vi "set offset.vi"(8 "error in (no error)":errorcluster, 11 "Thorcam in":refnum<class "Thorcam.lvclass">) -> (0 "error out":errorcluster, 3 "Thorcam out":refnum<class "Thorcam.lvclass">)   [LabVIEW 2012, in "Thorcam.lvclass"]
uses:
  Thorcam.lvclass
  Thorcam.lvclass/Thorcam.ctl
panel:
  out "Value":i32
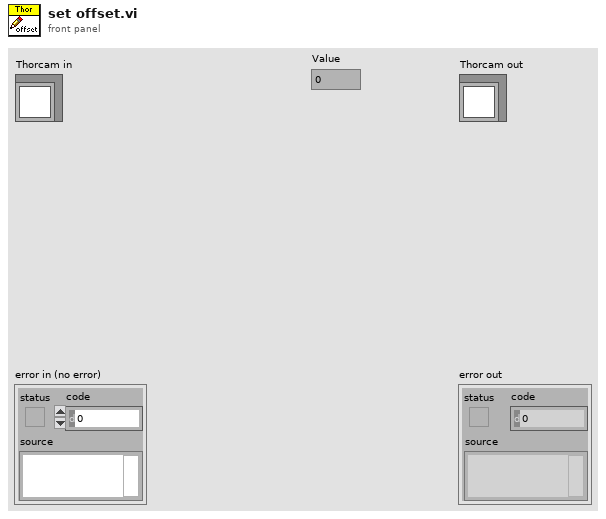
[diagram p1: front panel]
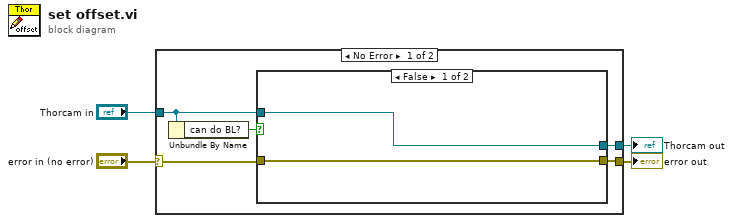
[diagram p0: block diagram]
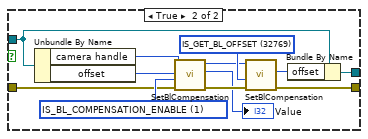
[diagram p2: hidden frame]
diagram:
  n1 = case shown="No Error" "error in (no error)" {
    selector: "error in (no error)" -> [w9 w25]
    tunnel: [w6 w25] -> w3
    tunnel: [w5 w24] -> w1
    tunnel: "Thorcam in" -> [w8 w24]
    frame No Error {
      n2 = Unbundle By Name(w8) -> ("can do BL?"=w7:bool)
      n3 = case shown="False" w7 {
        tunnel: w8 -> [w11 w14]
        tunnel: w9 -> [w10 w21]
        tunnel: [w10 w18] -> w6
        tunnel: [w11 w13] -> w5
        frame False {
        }
        frame True {
          w17 = 32769 items=["IS_BL_COMPENSATION_DISABLE"=0, "IS_BL_COMPENSATION_ENABLE"=1, "IS_GET_BL_COMPENSATION"=32768, "IS_GET_BL_OFFSET"=32769, "IS_GET_BL_DEFAULT_MODE"=32770, "IS_GET_BL_DEFAULT_OFFSET"=32771, "IS_GET_BL_SUPPORTED_MODE"=32772, "IS_IGNORE_PARAMETER"=-1] ("Mode")
          w23 = 1 items=["IS_BL_COMPENSATION_DISABLE"=0, "IS_BL_COMPENSATION_ENABLE"=1, "IS_GET_BL_COMPENSATION"=32768, "IS_GET_BL_OFFSET"=32769, "IS_GET_BL_DEFAULT_MODE"=32770, "IS_GET_BL_DEFAULT_OFFSET"=32771, "IS_GET_BL_SUPPORTED_MODE"=32772, "IS_IGNORE_PARAMETER"=-1] ("Mode")
          n4 = Unbundle By Name(w14) -> ("camera handle"=w22:u32, "offset"=w20:i32)
          n5 = call <instrlib>:"SetBlCompensation.vi"("error in"=w21, "Mode"=w23, "offset"=w20, "Camera Handle In"=w22) -> ("error out"=w19:errorcluster, "Value"=→"Value":i32, "Camera Handle Out"=w16:u32)  [unwired: 5 in]
          n6 = call <instrlib>:"SetBlCompensation.vi"("error in"=w19, "Mode"=w17, "Camera Handle In"=w16) -> ("error out"=w18:errorcluster, "Value"=w15:i32)  [unwired: 6 in, 1 out]
          n7 = Bundle By Name(cluster=w14, "offset"=w15) -> (w13:refnum<class "Thorcam.lvclass">)
        }
      }
    }
    frame Error {
    }
  }
  "error out" <- w3
  "Thorcam out" <- w1
